vi "Scan for Hardware.vi"(8 "error in (no error)":errorcluster, 11 "Mag Lab Measure Controller in":refnum<class "Mag Lab Measure Controller.lvclass">) -> (0 "error out":errorcluster, 3 "Mag Lab Measure Controller out":refnum<class "Mag Lab Measure Controller.lvclass">)   [LabVIEW 2015, in "Mag Lab Measure Controller.lvclass"]
uses:
  Mag Lab Measure Controller.lvclass
  Hardware/Mag Lab Hardware.lvclass
panel:
  out "VI Path":path
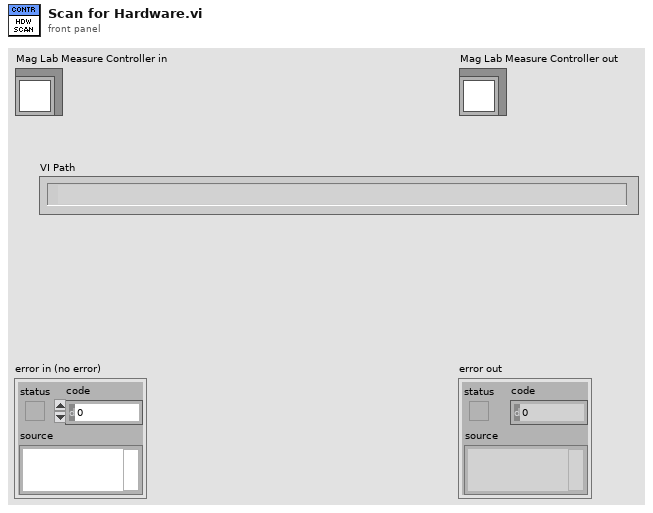
[diagram p1: front panel]
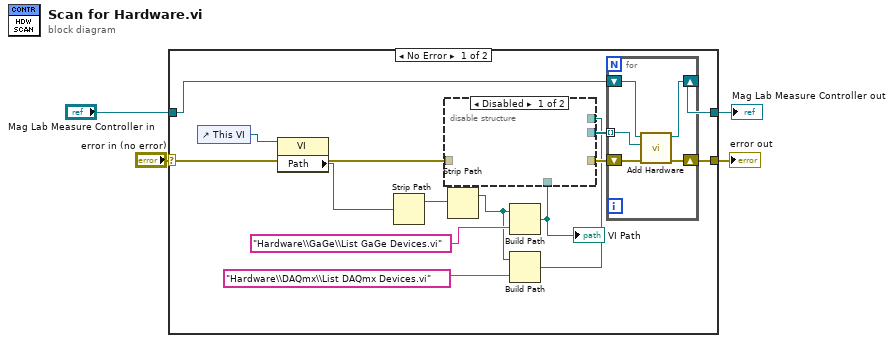
[diagram p0: block diagram]
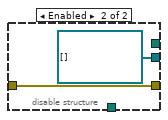
[diagram p2: hidden frame]
diagram:
  n1 = case shown="No Error" "error in (no error)" {
    selector: "error in (no error)" -> [w18 w27]
    tunnel: [w13 w27] -> w3
    tunnel: [w14 w26] -> w1
    tunnel: "Mag Lab Measure Controller in" -> [w17 w26]
    frame No Error {
      n2 = control-ref of="This VI"() -> (w12:refnum<vi>)
      n3 = property class="VI"(reference=w12) -> ("Path"=w11:path)  [unwired: 1 in, 2 out]
      n4 = Strip Path(path=w11) -> (stripped path=w10:path)  [unwired: 1 out]
      n5 = Strip Path(path=w10) -> (stripped path=w7:path)  [unwired: 1 out]
      n6 = Build Path(base path=w7, name or relative path="Hardware\\GaGe\\List GaGe Devices.vi") -> (appended path=w5:path)
      "VI Path" <- w5
      n7 = Build Path(base path=w7, name or relative path="Hardware\\DAQmx\\List DAQmx Devices.vi") -> (appended path=w6:path)
      n8 = disable-structure shown="Disabled" {
        disable-tunnel: w18 -> [_ w20]
        disable-tunnel: [_ refnum<class "Mag Lab Hardware.lvclass">[] []] -> w16
        disable-tunnel: [_ w20] -> w15
        disable-tunnel: w6 -> [_ _]
        disable-tunnel: w5 -> [_ _]
        frame Disabled {
        }
        frame Enabled {
        }
      }
      n9 = for {
        shift-right: [w24] -> w14
        shift-left: w17 -> [w25]
        tunnel: w16 -> [w23] mode=indexing
        shift-right: [w21] -> w13
        shift-left: w15 -> [w22]
        n10 = call-dynamic "Add Hardware.vi"("error in (no error)"=w22, "Mag Lab Hardware.lvclass"=w23, "Mag Lab Measure Controller in"=w25) -> ("error out"=w21:errorcluster, "Mag Lab Measure Controller out"=w24:refnum<class "Mag Lab Measure Controller.lvclass">)  [unwired: 7 in]
      }
    }
    frame Error {
    }
  }
  "error out" <- w3
  "Mag Lab Measure Controller out" <- w1
